vi "Position calling vi to LR 2.vi"(3 "error in (no error)":errorcluster, 4 "Corner":enum16{"LR", "LL"}(ring)) -> (0 "error out":errorcluster, 2 "call chain":string[](array[string]))   [LabVIEW 2016]
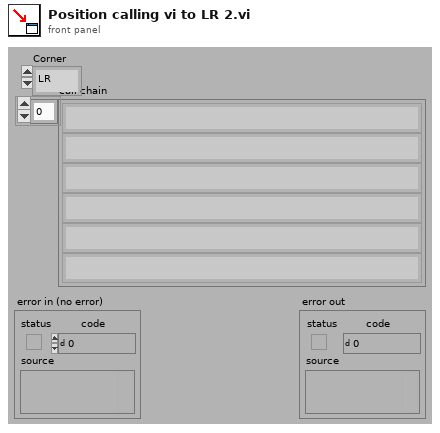
[diagram p1: front panel]
types:
  T1 = typedef "LVRectTypeDef.ctl" = cluster{"Left":i16, "Top":i16, "Right":i16, "Bottom":i16}
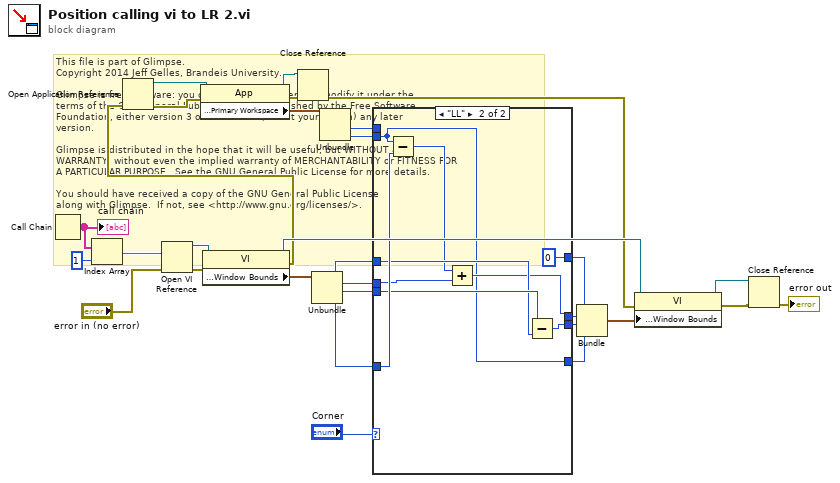
[diagram p0: block diagram]
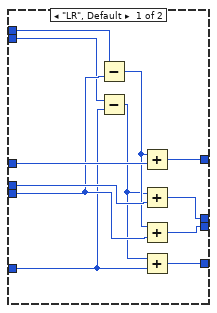
[diagram p2: hidden frame]
diagram:
  # "This file is part of Glimpse. \nCopyright 2014 Jeff Gelles, Brandeis University.    \n\nGlimpse is free software: you can redistribute it and/or modify it under the \nterms of the GNU General Public License as published by the Free Software \nFoundation, either version 3 of the License, or (at your option) any later \nversion.\n\nGlimpse is distributed in the hope that it will be useful, but WITHOUT ANY \nWARRANTY; without even the implied warranty of MERCHANTABILITY or FITNESS FOR \nA PARTICULAR PURPOSE.  See the GNU General Public License for more details.\n\nYou should have received a copy of the GNU General Public License\nalong with Glimpse.  If not, see <http://www.gnu.org/licenses/>."
  n1 = Call Chain() -> (call chain=w30:string[])
  "call chain" <- w30
  n2 = Index Array(array=w30, index=1 ("Index")) -> (element=w28:string)
  n3 = Open VI Reference(vi path=w28, error in (no error)="error in (no error)") -> (vi reference=w27:refnum<vi>, error out=w26:errorcluster)  [unwired: 4 out]
  n4 = property class="VI"(reference=w27, error in=w26) -> (reference out=w14:refnum<vi>, error out=w5:errorcluster, "Front Panel Window:Window Bounds"=w25:T1)
  n5 = Open Application Reference(8:w5) -> (0:w4:errorcluster, 3:w10:refnum<vi>)  [unwired: 3 out]
  n6 = property class="App"(reference=w10, error in=w4) -> (reference out=w2:refnum<vi>, error out=w6:errorcluster, "Display:Primary Workspace"=w9:T1)
  n7 = Close Reference(reference=w2, error in (no error)=w6) -> (error out=w3:errorcluster)
  n8 = Unbundle(w25) -> ("Left"=w23:i16, "Top"=w22:i16, "Right"=w21:i16, "Bottom"=w20:i16)
  n9 = Unbundle(w9) -> ("Right"=w8:i16, "Bottom"=w7:i16)  [unwired: 2 out]
  n10 = case shown="\"LL\"" "Corner" {
    tunnel: w23 -> [w42 w47]
    tunnel: w22 -> [w41 w45]
    tunnel: w21 -> [w40 w48]
    tunnel: w20 -> [w38 w51]
    tunnel: [w36 w43] -> w18
    tunnel: [w35 i16 0] -> w17
    tunnel: [w34 w49] -> w16
    tunnel: [w33 w44] -> w15
    tunnel: w8 -> [w32 _]
    tunnel: w7 -> [w31 w43]
    frame "LR", Default {
      n11 = Subtract(x=w32, y=w40) -> (x-y=w39:i16)
      n12 = Subtract(x=w31, y=w38) -> (x-y=w37:i16)
      n13 = Add(x=w39, y=w42) -> (x+y=w35:i16)
      n14 = Add(x=w37, y=w41) -> (x+y=w33:i16)
      n15 = Add(x=w39, y=w40) -> (x+y=w34:i16)
      n16 = Add(x=w37, y=w38) -> (x+y=w36:i16)
    }
    frame "LL" {
      n17 = Subtract(x=w43, y=w51) -> (x-y=w46:i16)
      n18 = Add(x=w46, y=w45) -> (x+y=w44:i16)
      n19 = Subtract(x=w48, y=w47) -> (x-y=w49:i16)
    }
  }
  n20 = Bundle(w17, w15, w16, "Bottom"=w18) -> (w19:cluster{i16, i16, i16, "Bottom":i16})  [unwired: 1 out]
  n21 = property class="VI"(reference=w14, error in=w3, "Front Panel Window:Window Bounds"=w19) -> (reference out=w12:refnum<vi>, error out=w13:errorcluster)
  n22 = Close Reference(reference=w12, error in (no error)=w13) -> (error out=→"error out":errorcluster)
